vi "Data JSON.vi"(8 "error in (no error)":errorcluster, 11 "Client Message in":refnum<class "Client Message.lvclass">) -> (0 "error out":errorcluster, 2 "Data JSON":string, 3 "Client Message out":refnum<class "Client Message.lvclass">)   [LabVIEW 2020, in "obs-websocket.lvlib" / "Client Message.lvclass"]
uses:
  Client Message.lvclass
  Client Message.lvclass/Client Message.ctl
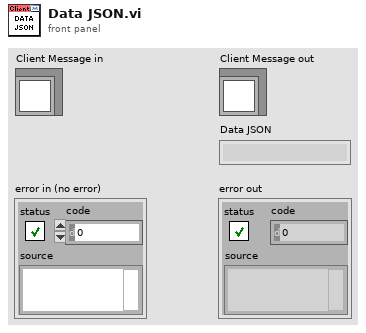
[diagram p1: front panel]
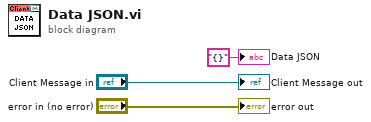
[diagram p0: block diagram]
diagram:
  "error out" <- "error in (no error)"
  "Client Message out" <- "Client Message in"
  "Data JSON" <- "{}" ("Data JSON")
